vi "加速度_脉冲指标.vi"(10 "峰值":dbl, 11 "信号X":dbl[](array[numeric])) -> (3 "脉冲指标":dbl)   [LabVIEW 2014]
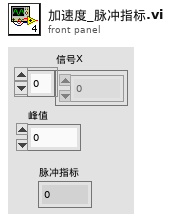
[diagram p1: front panel]
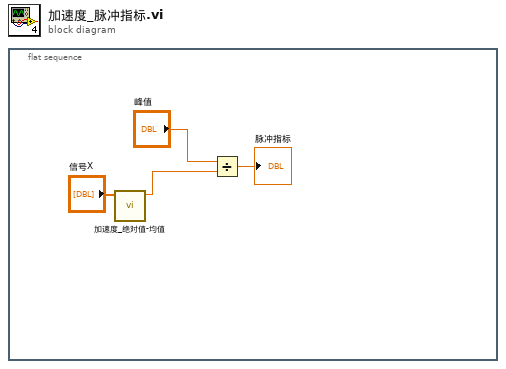
[diagram p0: block diagram]
diagram:
  n1 = flat-sequence {
    frame #0 {
      n2 = call "加速度_绝对值-均值.vi"("信号X"="信号X") -> ("均值"=w3:dbl)  [unwired: 10 in]
      n3 = Divide(x="峰值", y=w3) -> (x/y=→"脉冲指标":dbl)
    }
  }
